vi "PC_Main.vi"() -> ()   [LabVIEW 2015]
uses:
  <vilib>/vision/driver/NI_Vision_Acquisition_Software.lvlib
  <vilib>/vision/NI_Vision_Development_Module.lvlib
  <vilib>/userdefined/High Color/IMAQdx.ctl
panel:
  in  "Number of Erosion":i32=6
  in  "Range":cluster{"Lower value":sgl, "Upper value":sgl}={"Lower value"=128.0, "Upper value"=255.0} {"Upper value" format="%.2f"; "Lower value" format="%.2f"}
  in  "Color Plane":i32(ring)=1 items=["Red", "Green", "Blue", "Hue", "Saturation", "Luminance", "Value", "Intensity"]
  in  "File Path":path=path "\\\\hs7.lboro.ac.uk\\mmsc4/GitHub/mechatronics/LabVIEW/calibration6.png"
  in  "Angle (degrees)":sgl format="%.2f"
  in  "Mirror":bool=TRUE
  in  "Symmetry":u32(ring)=1 items=["Horizontal", "Vertical", "Central", "1st Diagonal", "2nd Diagonal"]
  in  "Camera":T1="cam1"
  out "Image":T2(plugin-control)
  in  "stop":bool
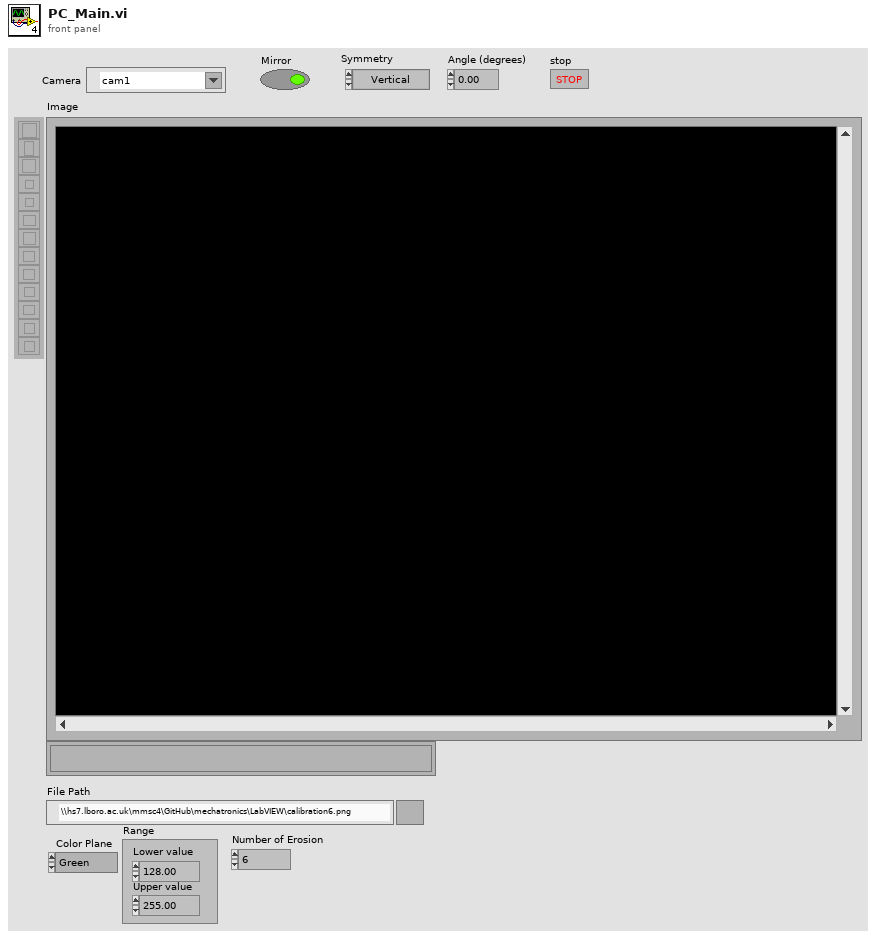
[diagram p1: front panel]
types:
  T1 = typedef "IMAQdx.ctl" = refnum<k21>
  T2 = typedef "IMAQ Image.ctl" = refnum<image>
  T3 = typedef "Image Type" = u32
  T4 = enum8{"Enabled", "Disabled", "Disabled and Grayed Out"}
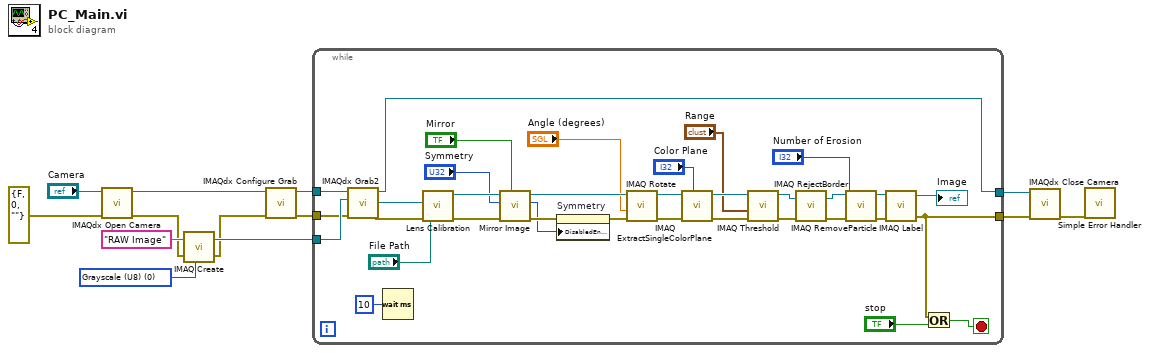
[diagram p0: block diagram]
diagram:
  w8 = T3 0 items=["Grayscale (U8)", "Grayscale (I16)", "Grayscale (SGL)", "Complex (CSG)", "RGB (U32)", "HSL (U32)", "RGB (U64)", "Grayscale (U16)"] ("Image Type")
  n1 = call <vilib>:"IMAQdx Open Camera.vi"("error in"=errorcluster {"status"=FALSE, "code"=0, "source"=""}, "Session In"="Camera") -> ("error out"=w5:errorcluster, "Session Out"=w13:T1)  [unwired: 8 in]
  n2 = call "IMAQ Create"("Image Name"="RAW Image", "Image Type"=w8, "error in (no error)"=w5) -> ("New Image"=w10:T2, "error out"=w4:errorcluster)  [unwired: 2 in]
  n3 = call <vilib>:"IMAQdx Configure Grab.vi"("error in"=w4, "Session In"=w13) -> ("error out"=w11:errorcluster, "Session Out"=w12:T1)  [unwired: 8 in]
  n4 = while {
    tunnel: w12 -> [w47]
    tunnel: w11 -> [w45]
    tunnel: w10 -> [w46]
    tunnel: [w42] -> w6
    tunnel: [w14] -> w2
    stop <- w44 stop-if-true
    n5 = call <vilib>:"IMAQdx Grab2.vi"("error in"=w45, "Image In"=w46, "Session In"=w47) -> ("error out"=w38:errorcluster, "Image Out"=w40:T2, "Session Out"=w42:T1)  [unwired: 5 in, 1 out]
    n6 = Wait (ms)(milliseconds to wait=u32 10) -> ()  [unwired: 1 out]
    n7 = call "Lens Calibration.vi"("Error In"=w38, "File Path"="File Path", "Image In"=w40) -> ("error out"=w37:errorcluster, "Image Out"=w41:T2)  [unwired: 3 in]
    n8 = call "Mirror Image.vi"("Mirror"="Mirror", "error in (no error)"=w37, "Symmetry"="Symmetry", "Refnum in"=w41) -> ("error out"=w33:errorcluster, "Disabled"=w31:T4, "Refnum out"=w36:T2)  [unwired: 5 in]
    n9 = property on="Symmetry" class="Ring (strict)"(error in=w33, "DisabledEnum"=w31) -> (error out=w32:errorcluster)  [unwired: 1 in, 1 out]
    n10 = call "IMAQ Rotate"("error in (no error)"=w32, "Angle (degrees)"="Angle (degrees)", "Image Src"=w36) -> ("error out"=w28:errorcluster, "Image Dst Out"=w29:T2)  [unwired: 7 in]
    n11 = call "IMAQ ExtractSingleColorPlane"("Color Plane"="Color Plane", "error in (no error)"=w28, "Image Src"=w29) -> ("error out"=w25:errorcluster, "Image Dst Out"=w26:T2)  [unwired: 7 in]
    n12 = call "IMAQ Threshold"("error in (no error)"=w25, "Range"="Range", "Image Src"=w26) -> ("error out"=w21:errorcluster, "Image Dst Out"=w22:T2)  [unwired: 7 in]
    n13 = call "IMAQ RejectBorder"("error in (no error)"=w21, "Image Src"=w22) -> ("error out"=w19:errorcluster, "Image Dst Out"=w20:T2)  [unwired: 4 in]
    n14 = call "IMAQ RemoveParticle"("error in (no error)"=w19, "Number of Erosion"="Number of Erosion", "Image Src"=w20) -> ("error out"=w17:errorcluster, "Image Dst Out"=w16:T2)  [unwired: 7 in]
    n15 = call "IMAQ Label"("error in (no error)"=w17, "Image Src"=w16) -> ("error out"=w14:errorcluster, "Image Dst Out"=→"Image":T2)  [unwired: 2 in, 1 out]
    n16 = Or(x=w14, y="stop") -> (x .or. y?=w44:bool)
  }
  n17 = call <vilib>:"IMAQdx Close Camera.vi"("error in"=w2, "Session In"=w6) -> ("error out"=w1:errorcluster)  [unwired: 9 in]
  n18 = call <vilib>:"Simple Error Handler.vi"("error in (no error)"=w1) -> ()  [unwired: 4 in, 5 out]
